vi "Inficon - Reset XTC2.vi"(8 "Error In":errorcluster, 11 "COM port in":refnum<visa-resource-name>) -> (0 "Error Out":errorcluster, 3 "COM port out":refnum<visa-resource-name>)   [LabVIEW 2014]
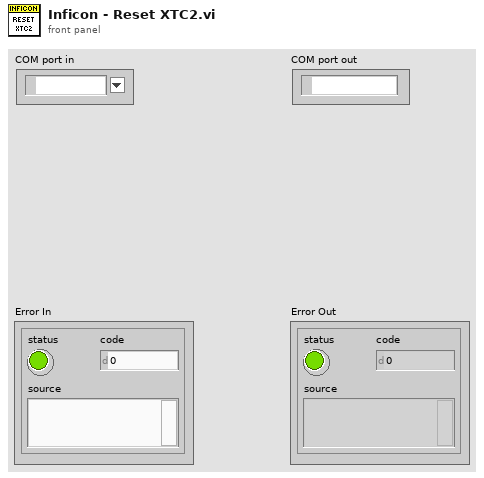
[diagram p1: front panel]
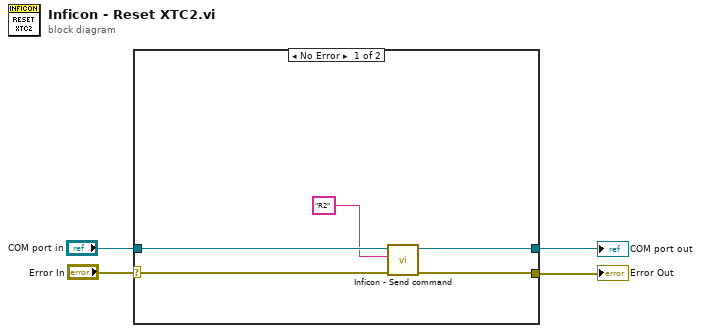
[diagram p0: block diagram]
diagram:
  n1 = case shown="No Error" "Error In" {
    selector: "Error In" -> [w9 w11]
    tunnel: [w8 w11] -> w3
    tunnel: "COM port in" -> [w7 w10]
    tunnel: [w6 w10] -> w1
    frame No Error {
      n2 = call "Inficon - Send command.vi"("Error In"=w9, "Command"="R2", "COM in"=w7) -> ("Error Out"=w8:errorcluster, "COM out"=w6:refnum<visa-resource-name>)  [unwired: 6 in, 1 out]
    }
    frame Error {
    }
  }
  "Error Out" <- w3
  "COM port out" <- w1
